vi "Interface.vi"(9 "UUT Result":refnum<user-event>, 10 "Exit":refnum<user-event>, 11 "VI ref":refnum<notifier>) -> ()   [LabVIEW 2019, in "Test Unit.lvlib"]
uses:
  Test Unit.lvlib
  UUT Result.ctl
  <vilib>/Test Bench Framework/Test Executive.lvlibp/TestEngine/TestEngine/TestEngine/Typedefs/Report General.ctl
  <vilib>/Test Bench Framework/Test Executive.lvlibp/TestEngine/TestEngine/TestEngine/Test Engine.lvclass
panel:
  in  "UUT State":string
  in  "SerialNumber":string
  in  "Cycle Time":string
  in  "Yields":dbl format="%.2f%%"
  in  "Failed":u32
  in  "Totals":u32 format="Total: %d"
  in  "Tree":string(tree)
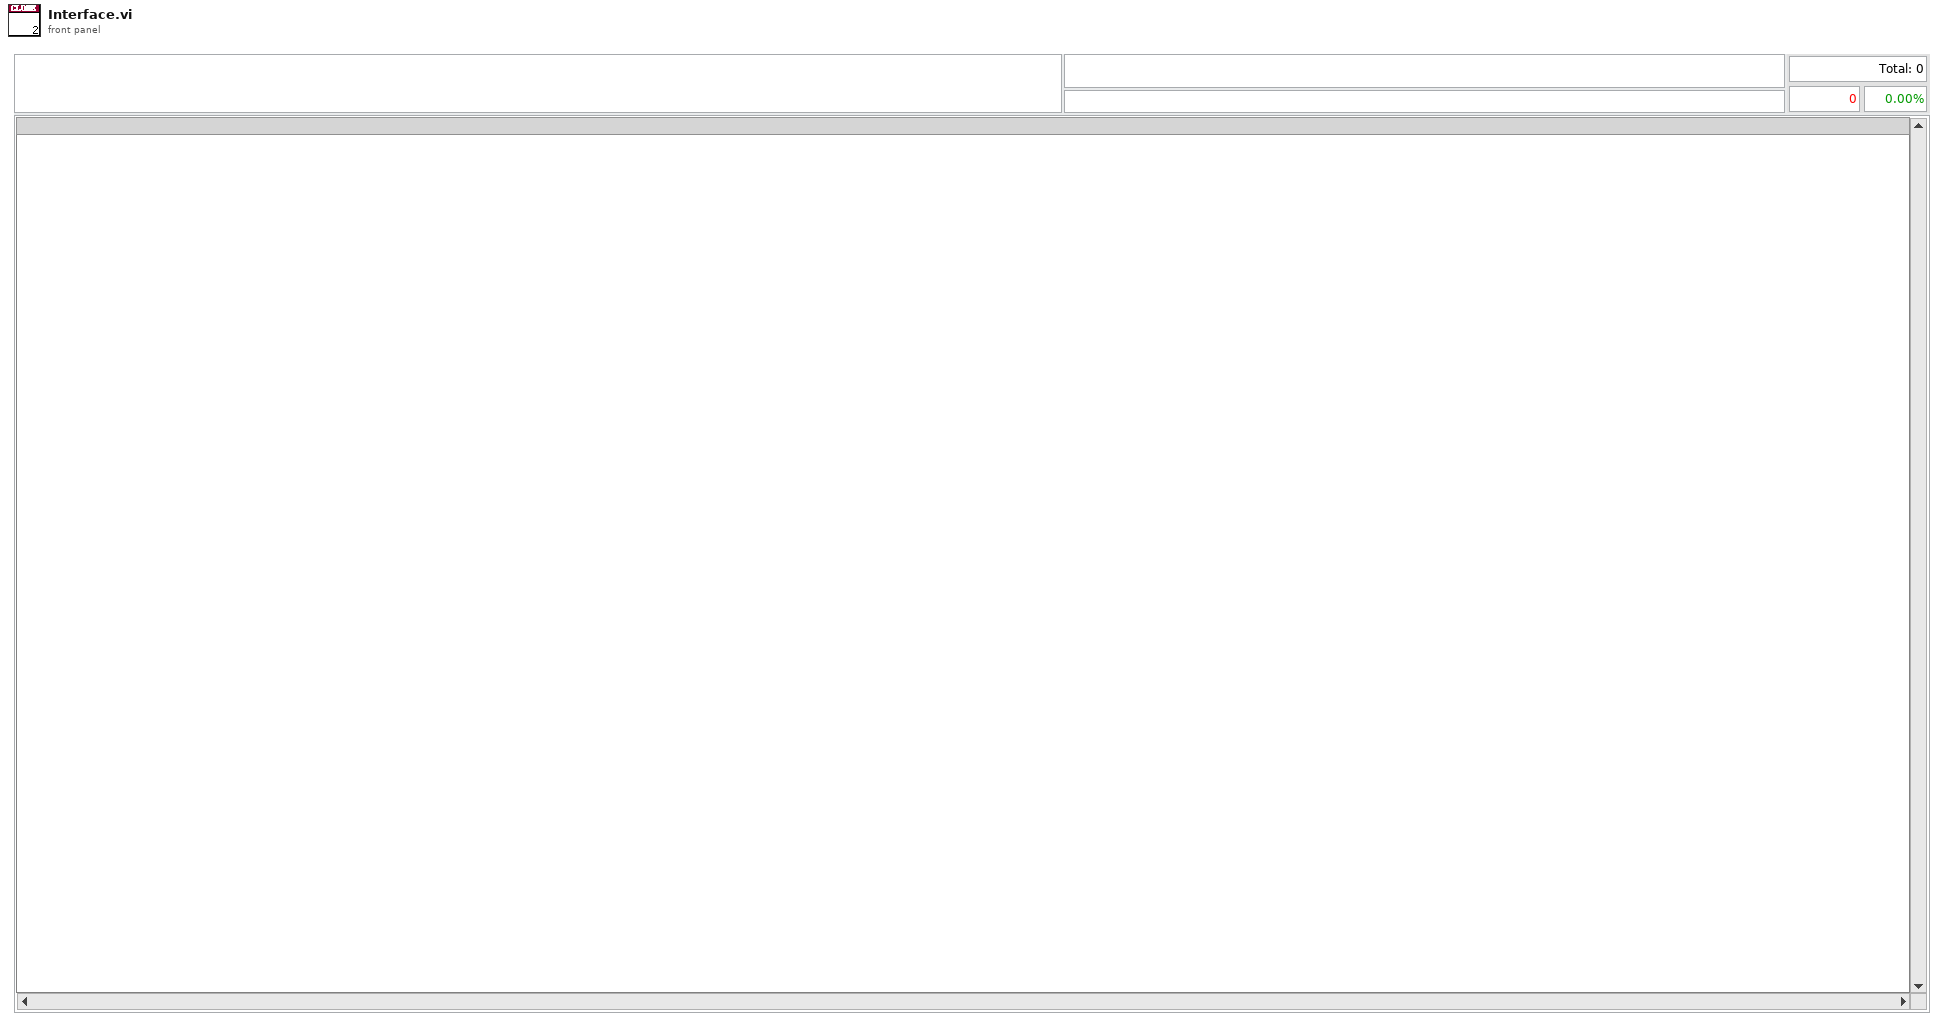
[diagram p1: front panel]
types:
  T1 = cluster{"Station":i32, "Socket":i32, "Sequence Path":path, "UUT Status":string}
  T2 = cluster{"UUT State":refnum<vi>, "Cycle Time":refnum<vi>, "SerialNumber":refnum<vi>, "Tree":refnum<vi>, "This VI":refnum<vi>}
  T3 = cluster{"Totals":refnum<vi>, "Failed":refnum<vi>, "Yields":refnum<vi>}
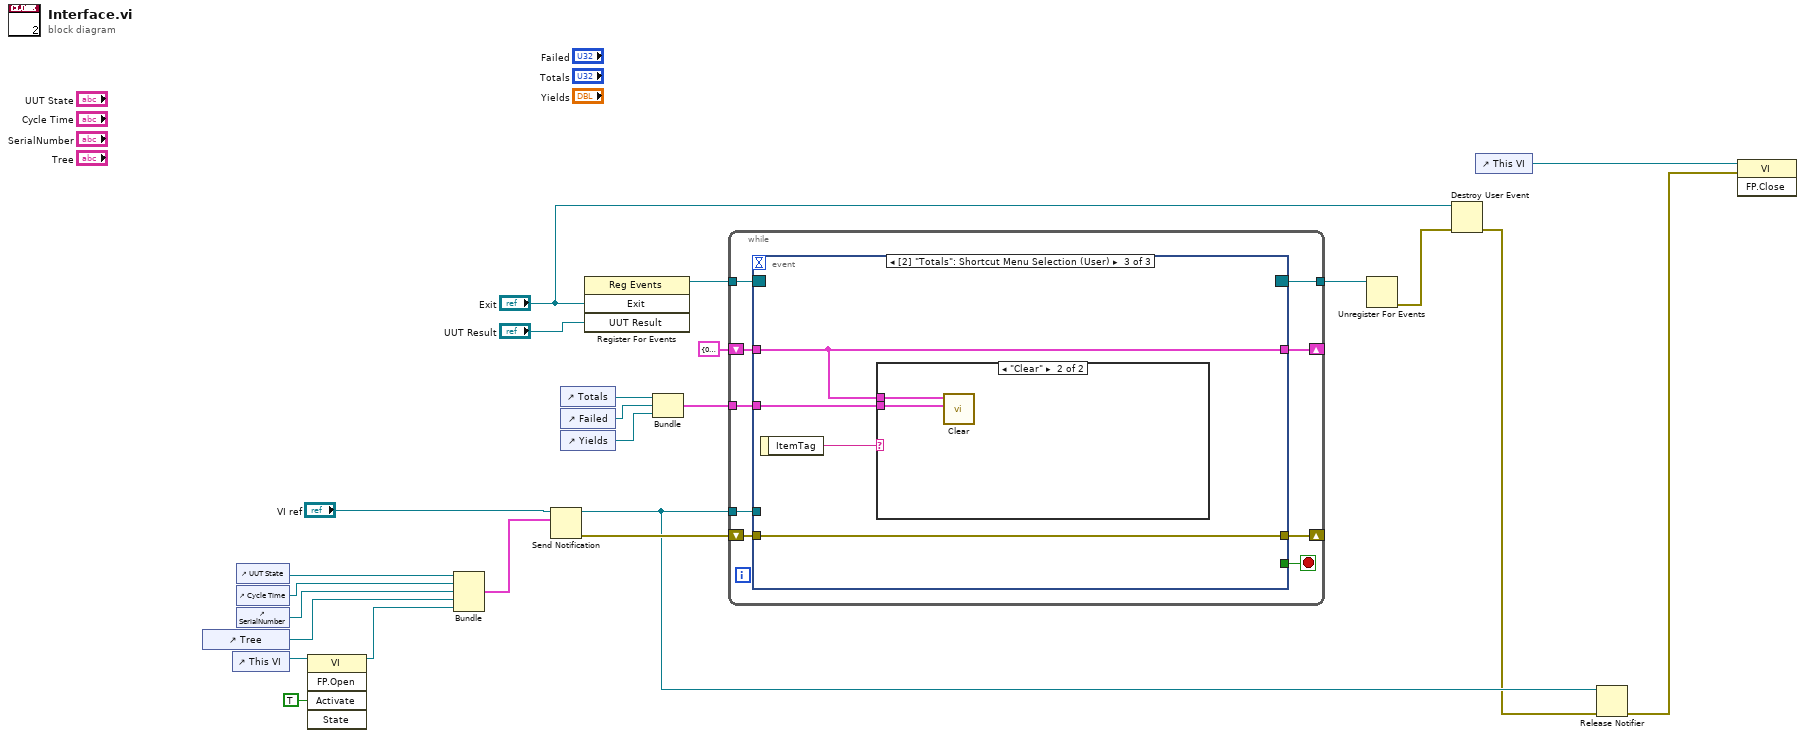
[diagram p0: block diagram]
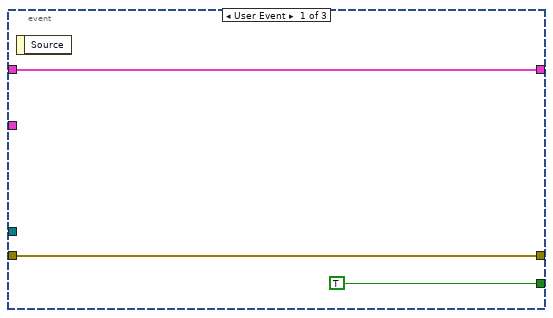
[diagram p2: hidden frame]
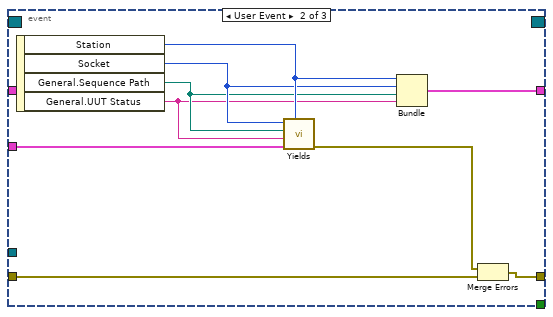
[diagram p3: hidden frame]
diagram:
  n1 = control-ref of="Tree"() -> (w19:refnum<vi>)
  n2 = control-ref of="This VI"() -> (w24:refnum<vi>)
  n3 = control-ref of="UUT State"() -> (w22:refnum<vi>)
  n4 = control-ref of="Cycle Time"() -> (w21:refnum<vi>)
  n5 = control-ref of="SerialNumber"() -> (w20:refnum<vi>)
  n6 = invoke class="VI" method="FP.Open"(reference=w24, "Activate"=TRUE ("Activate?")) -> (reference out=w18:refnum<vi>)  [unwired: 3 in, 4 out]
  n7 = Bundle("UUT State"=w22, "Cycle Time"=w21, "SerialNumber"=w20, "Tree"=w19, "This VI"=w18) -> (w13:T2)  [unwired: 1 in]
  n8 = Send Notification(notification=w13, notifier="VI ref") -> (notifier out=w10:refnum<notifier>, error out=w12:errorcluster)  [unwired: 1 in]
  n9 = control-ref of="Totals"() -> (w5:refnum<vi>)
  n10 = control-ref of="Failed"() -> (w4:refnum<vi>)
  n11 = control-ref of="Yields"() -> (w3:refnum<vi>)
  n12 = register-events("Exit", "UUT Result") -> (reference out=w17:refnum<event-registration>)  [unwired: 2 in, 1 out]
  n13 = Bundle("Totals"=w5, "Failed"=w4, "Yields"=w3) -> (w2:T3)  [unwired: 1 in]
  n14 = while {
    tunnel: w17 -> [w33]
    tunnel: [w31] -> w16
    tunnel: w10 -> [w30]
    shift-right: [w28] -> _
    shift-left: w12 -> [w29]
    tunnel: w2 -> [w27]
    shift-right: [w26] -> _
    shift-left: T1 {"Station"=0, "Socket"=0, "Sequence Path"=path "", "UUT Status"=""} -> [w25]
    stop <- w32 stop-if-true
    n15 = event shown="[2] \"Totals\": Shortcut Menu Selection (User)" {
      selector: w33 -> [_ _ _]
      dyn-events: [_ _ _] -> w31
      timeout: _ -> [_ _ _]
      tunnel: [TRUE _ _] -> w32
      tunnel: w30 -> [_ _ _]
      tunnel: w29 -> [w35 w44 w48]
      tunnel: [w35 w43 w48] -> w28
      tunnel: w27 -> [_ w45 w46]
      tunnel: [w34 w37 w47] -> w26
      tunnel: w25 -> [w34 _ w47]
      event User Event {
        n16 = event-data() -> ()  [unwired: 1 in, 1 out]
      }
      event User Event {
        n17 = event-data() -> ("Station"=w41:i32, "Socket"=w40:i32, "General.Sequence Path"=w39:path, "General.UUT Status"=w38:string)  [unwired: 1 in]
        n18 = call "Yields.vi"("Station"=w41, "Control"=w45, "UUT State"=w38, "General.Sequence Path"=w39, "Socket"=w40) -> ("error out"=w42:errorcluster)  [unwired: 6 in]
        n19 = Bundle("Station"=w41, "Socket"=w40, "Sequence Path"=w39, "UUT Status"=w38) -> (w37:T1)  [unwired: 1 in]
        n20 = Merge Errors(w42, w44) -> (w43:errorcluster)
      }
      event "Totals": Shortcut Menu Selection (User) {
        n21 = event-data() -> ("ItemTag"=w49:string)  [unwired: 1 in]
        n22 = case shown="\"Clear\"" w49 {
          tunnel: w47 -> [_ w51]
          tunnel: w46 -> [_ w50]
          frame Default {
          }
          frame "Clear" {
            n23 = call "Clear.vi"("Control"=w50, "Cluster"=w51) -> ()  [unwired: 9 in, 1 out]
          }
        }
      }
    }
  }
  n24 = Unregister For Events(event registration refnum=w16) -> (error out=w15:errorcluster)  [unwired: 1 in]
  n25 = Destroy User Event(user event="Exit", error in=w15) -> (error out=w9:errorcluster)
  n26 = control-ref of="This VI"() -> (w8:refnum<vi>)
  n27 = Release Notifier(notifier=w10, error in (no error)=w9) -> (error out=w7:errorcluster)  [unwired: 1 in, 2 out]
  n28 = invoke class="VI" method="FP.Close"(reference=w8, error in=w7) -> ()  [unwired: 1 in, 3 out]
